vi "Read Montana Temp.vi"(6 "milliseconds to wait":u32=10, 7 "Maximum Trials":i32=3, 8 "error in":errorcluster, 10 "Command":string="03GPT", 11 "Address":string="10.0.0.3") -> (0 "error out":errorcluster, 2 "Current temp 2":dbl=5.585)   [LabVIEW 2025, in "MyMontana.lvlib"]
uses:
  MyMontana.lvlib
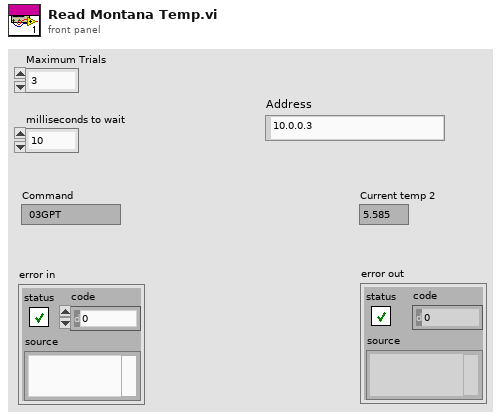
[diagram p1: front panel]
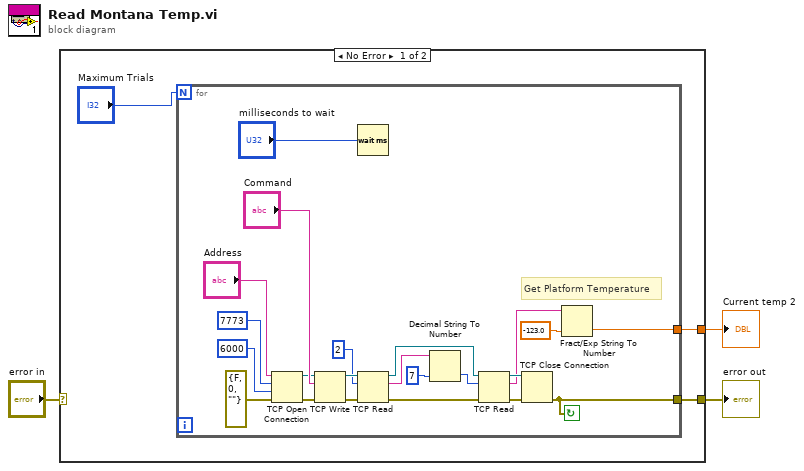
[diagram p0: block diagram]
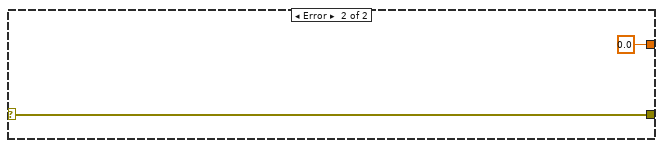
[diagram p2: hidden frame]
diagram:
  n1 = case shown="No Error" "error in" {
    selector: "error in" -> [_ w30]
    tunnel: [w6 w30] -> w3
    tunnel: [w5 0.0] -> w2
    frame No Error {
      n2 = for {
        N: "Maximum Trials" -> [_]
        tunnel: [w8] -> w5
        tunnel: [w7] -> w6
        stop <- w7 continue-if-true
        # "Get Platform Temperature"
        n3 = TCP Open Connection(address="Address", remote port or service name=u16 7773, timeout ms (60000)=6000, error in (no error)=errorcluster {"status"=FALSE, "code"=0, "source"=""}) -> (connection ID=w14:refnum<k5>, error out=w13:errorcluster)  [unwired: 1 in]
        n4 = TCP Write(connection ID=w14, data in="Command", error in (no error)=w13) -> (connection ID out=w24:refnum<k5>, error out=w18:errorcluster)  [unwired: 1 in, 1 out]
        n5 = Wait (ms)(milliseconds to wait="milliseconds to wait") -> ()  [unwired: 1 out]
        n6 = TCP Read(connection ID=w24, bytes to read=2, error in (no error)=w18) -> (connection ID out=w21:refnum<k5>, data out=w22:string, error out=w17:errorcluster)  [unwired: 2 in]
        n7 = Decimal String To Number(string=w22, default (0L)=7 ("default (0 I32)")) -> (number=w20:i32)  [unwired: 1 in, 1 out]
        n8 = TCP Read(connection ID=w21, bytes to read=w20, error in (no error)=w17) -> (connection ID out=w27:refnum<k5>, data out=w19:string, error out=w25:errorcluster)  [unwired: 2 in]
        n9 = TCP Close Connection(connection ID=w27, error in (no error)=w25) -> (error out=w7:errorcluster)  [unwired: 1 in, 1 out]
        n10 = Fract/Exp String To Number(string=w19, default (0 dbl)=-123.0 ("default (0 DBL)")) -> (number=w8:dbl)  [unwired: 2 in, 1 out]
      }
    }
    frame Error {
    }
  }
  "error out" <- w3
  "Current temp 2" <- w2
